vi "OutbitsGlobalVars.vi"() -> ()   [LabVIEW 2014]
uses:
  OutbitsStateControl.ctl
panel:
  in  "nOfCmdsOutbit2":u32
  in  "nOfCmdsOutbit1":u32
  in  "nOfCmdsOutbit0":u32
  out "OutBitStopListening":bool
  in  "OutBitsState":T1
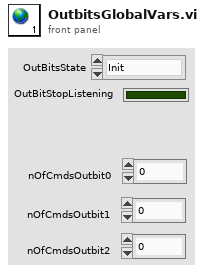
[diagram p1: front panel]
types:
  T1 = typedef "OutbitsStateControl.ctl" = enum16{"Init", "Idle", "loading", "listening", "clearing", "error"}
diagram:
